vi "Actor Core.vi"(8 "error in":errorcluster, 11 "ResultsViewer in":refnum<class "ResultsViewer.lvclass">) -> (0 "error out":errorcluster, 3 "Actor out":refnum<class "Actor.lvclass">)   [LabVIEW 2019, in "ResultsViewer.lvlib" / "ResultsViewer.lvclass"]
doc: "(<B>Filename</B>: Actor Framework.lvlib:Actor.lvclass:Actor Core.vi)\n\nReceives messages to the actor, reacts to them, and initiates any error handling that may shut the actor down.\n\nDescendant classes may override this VI to append parallel tasks for the actor to complete while it handles messages. Overrides use the Call Parent Class Method node."
uses:
  ResultsViewer.lvclass
  C:/Program Files (x86)/National Instruments/LabVIEW 2019/vi.lib/ActorFramework/Actor/Actor.lvclass
  <vilib>/ActorFramework/Actor/Actor.lvclass
  ResultsViewer.lvclass/ResultsViewer.ctl
  <vilib>/ActorFramework/Actor/Actor.lvclass/Actor.ctl
  <vilib>/ActorFramework/Message Enqueuer/Message Enqueuer.lvclass/Message Enqueuer.ctl
  <vilib>/ActorFramework/Message Enqueuer/Init from Existing Queue.vi
  <vilib>/ActorFramework/Message Enqueuer/Enqueue.vi
  <vilib>/ActorFramework/Stop Msg/Stop Msg.lvclass
  C:/Program Files (x86)/National Instruments/LabVIEW 2019/vi.lib/ActorFramework/Message/Message.lvclass
  <vilib>/ActorFramework/Message Priority Queue/Priority Enqueue.vi
  <vilib>/ActorFramework/Message Enqueuer/Message Enqueuer.lvclass
panel:
  out "Loaded TDMS Filename":string
  out "O2 Saturation":dbl[](graph)
  out "Heart beat":dbl[](graph)
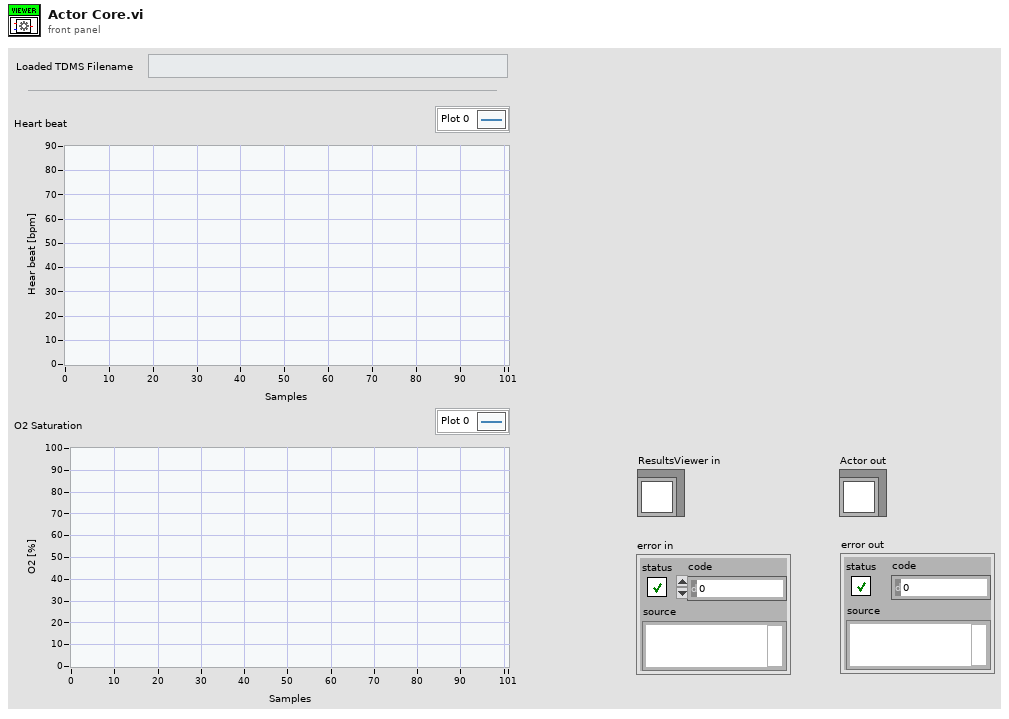
[diagram p1: front panel]
types:
  T1 = enum32{"Invalid", "Standard", "Closed", "Hidden", "Minimized", "Maximized"}
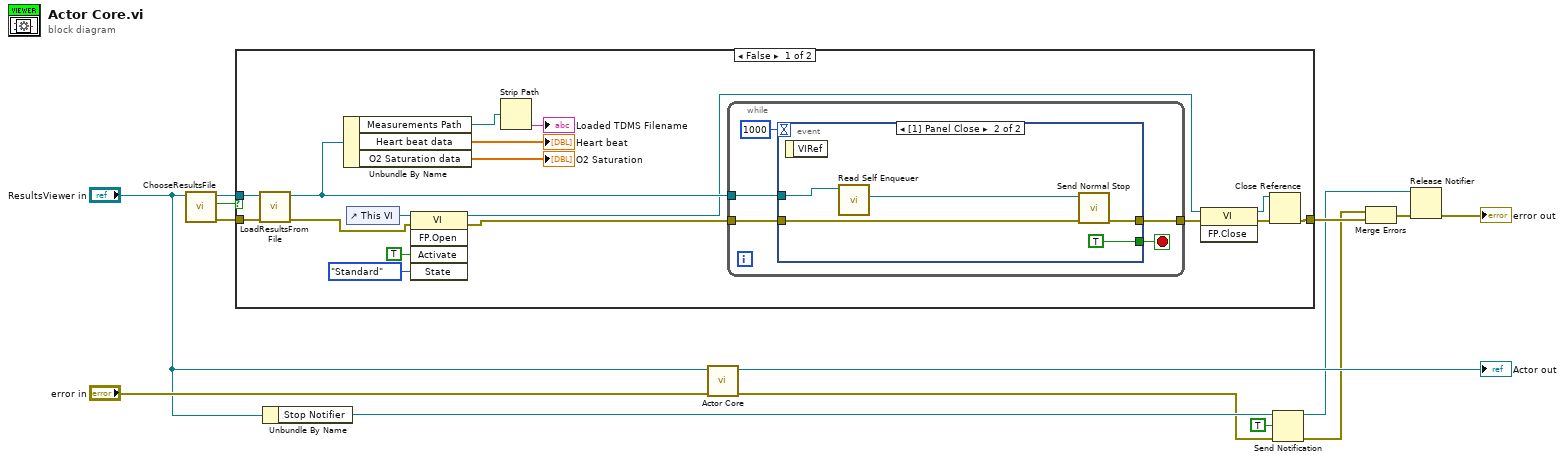
[diagram p0: block diagram]
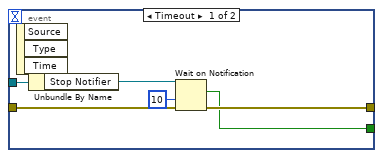
[diagram p2: hidden frame]
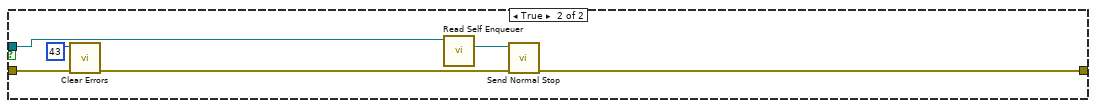
[diagram p3: hidden frame]
diagram:
  n1 = call "ChooseResultsFile.vi"("ResultsViewer in"="ResultsViewer in") -> ("error out"=w12:errorcluster, "Cancelled?"=w11:bool, "ResultsViewer out"=w13:refnum<class "ResultsViewer.lvclass">)  [unwired: 8 in]
  n2 = case shown="False" w11 {
    tunnel: w13 -> [w31 w52]
    tunnel: w12 -> [w30 w50]
    tunnel: [w16 w51] -> w10
    frame False {
      n3 = call "LoadResultsFromFile.vi"("error in (no error)"=w30, "ResultsViewer in"=w31) -> ("error out"=w21:errorcluster, "ResultsViewer out"=w29:refnum<class "ResultsViewer.lvclass">)  [unwired: 8 in]
      n4 = Unbundle By Name(w29) -> ("Measurements Path"=w26:path, "Heart beat data"=→"Heart beat":dbl[], "O2 Saturation data"=→"O2 Saturation":dbl[])
      n5 = control-ref of="This VI"() -> (w24:refnum<vi>)
      n6 = invoke class="VI" method="FP.Open"(reference=w24, error in=w21, "Activate"=TRUE ("Activate?"), "State"=T1."Standard") -> (reference out=w17:refnum<vi>, error out=w20:errorcluster)  [unwired: 1 in, 3 out]
      n7 = Strip Path(path=w26) -> (name=→"Loaded TDMS Filename":string)  [unwired: 1 out]
      n8 = while {
        tunnel: w20 -> [w35]
        tunnel: w29 -> [w36]
        tunnel: [w34] -> w19
        stop <- w33 stop-if-true
        n9 = event shown="[1] Panel Close" {
          selector: _ -> [_ _]
          dyn-events: _ -> [_ _]
          timeout: 1000 -> [_ _]
          tunnel: w36 -> [w41 w45]
          tunnel: w35 -> [w42 w46]
          tunnel: [w40 w43] -> w34
          tunnel: [w38 TRUE] -> w33
          event Timeout {
            n10 = event-data() -> ()  [unwired: 1 in, 3 out]
            n11 = Unbundle By Name(w41) -> ("Stop Notifier"=w39:refnum<notifier>)
            n12 = Wait on Notification(notifier=w39, timeout in ms (-1)=10, error in (no error)=w42) -> (notification=w38:bool, error out=w40:errorcluster)  [unwired: 1 in, 2 out]
          }
          event Panel Close {
            n13 = event-data() -> ()  [unwired: 1 in, 1 out]
            n14 = call <vilib>:"Read Self Enqueuer.vi"("Actor"=w45) -> ("Self Enqueuer"=w44:refnum<class "Message Enqueuer.lvclass">)  [unwired: 10 in]
            n15 = call <vilib>:"Send Normal Stop.vi"("error in (no error)"=w46, "Message Enqueuer"=w44) -> ("error out"=w43:errorcluster)  [unwired: 9 in]
          }
        }
      }
      n16 = invoke class="VI" method="FP.Close"(reference=w17, error in=w19) -> (reference out=w15:refnum<vi>, error out=w18:errorcluster)  [unwired: 1 in, 1 out]
      n17 = Close Reference(reference=w15, error in (no error)=w18) -> (error out=w16:errorcluster)
    }
    frame True {
      n18 = call <vilib>:"Clear Errors.vi"("error in (no error)"=w50, "specific error code to clear (0: all)"=43) -> ("error out"=w49:errorcluster)  [unwired: 4 in, 1 out]
      n19 = call <vilib>:"Read Self Enqueuer.vi"("Actor"=w52) -> ("Self Enqueuer"=w53:refnum<class "Message Enqueuer.lvclass">)  [unwired: 10 in]
      n20 = call <vilib>:"Send Normal Stop.vi"("error in (no error)"=w49, "Message Enqueuer"=w53) -> ("error out"=w51:errorcluster)  [unwired: 9 in]
    }
  }
  n21 = Unbundle By Name("ResultsViewer in") -> ("Stop Notifier"=w5:refnum<notifier>)
  n22 = call-parent "Actor Core.vi"("error in"="error in", "Actor in"="ResultsViewer in") -> ("error out"=w3:errorcluster, "Actor out"=→"Actor out":refnum<class "Actor.lvclass">)  [unwired: 8 in]
  n23 = Send Notification(notification=TRUE, notifier=w5, error in (no error)=w3) -> (notifier out=w4:refnum<notifier>, error out=w2:errorcluster)
  n24 = Merge Errors(w2, w10) -> (w9:errorcluster)
  n25 = Release Notifier(notifier=w4, error in (no error)=w9) -> (error out=→"error out":errorcluster)  [unwired: 1 in, 2 out]
